vi "Init Phasor Explorer Settings.vi"(8 "error in (no error)":errorcluster) -> (0 "error out":errorcluster)   [LabVIEW 2019]
uses:
  Phasor Explorer Settings List.ctl
  Phasor Explorer Display Parameters.ctl
  Type of Series.ctl
  Phasor Explorer Phasor Parameters.ctl
  Phasor Calculation Type.ctl
  SEPL Type.ctl
  Phasor Explorer Decay Parameters.ctl
  IRF Model.ctl
  Phasor Explorer Gate Parameters.ctl
  Gate Type.ctl
  Type of User-defined Function.ctl
  Phasor Explorer Detector Parameters.ctl
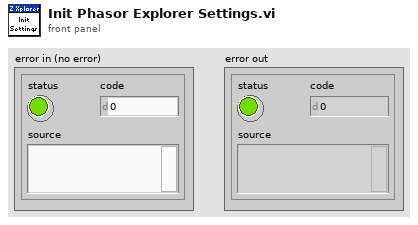
[diagram p1: front panel]
types:
  T1 = typedef "Phasor Explorer Settings List.ctl" = enum16{"Display Parameters", "Phasor Parameters", "Decay & IRF Parameters", "Gate Parameters", "Detector Parameters", "f*", "tau*"}
  T2 = typedef "Phasor Explorer Display Parameters.ctl" = cluster{"# Points":i32, "Ramp Type":enum16{"Linear", "Logarithmic"}, "Type of Series":T3, "Min tau":dbl[unit], "Max tau":dbl[unit], "Include 0":bool, "Include Infinity":bool}
  T3 = typedef "Type of Series.ctl" = enum16{"1-Exp Decays", "Linear Combination of 1-Exp"}
  T4 = typedef "Phasor Explorer Phasor Parameters.ctl" = cluster{"Harmonic Frequency":dbl[unit], "Use f* = 1/D Frequency":bool, "Calibrated Phasor":bool, "Calibration Lifetime":dbl[unit], "Phasor Calculation":T5, "SEPL Type":T6, "# Gates":dbl, "Square Gate Width":dbl[unit], "Show Ticks":bool}
  T5 = typedef "Phasor Calculation Type.ctl" = enum16{"Direct Sum", "Analytical Formula"}
  T6 = typedef "SEPL Type.ctl" = enum16{"UC", "L_N", "L_N[W]", "L_X"}
  T7 = typedef "Phasor Explorer Decay Parameters.ctl" = cluster{"Lifetime":dbl[unit], "IRF Offset":dbl[unit], "IRF Period":dbl[unit], "Normalized Decays":bool, "IRF Model":T8, "IRF Parameter 1":dbl[unit]}
  T8 = typedef "IRF Model.ctl" = enum16{"Dirac", "Exponential"}
  T9 = typedef "Phasor Explorer Gate Parameters.ctl" = cluster{"First Gate Start":dbl[unit], "Use Gate Center":bool, "Gate Width":dbl[unit], "Gate Step":dbl[unit], "# Gates":dbl, "Gate Type":T10, "Edge Width":dbl[unit], "Top Slope":dbl[unit], "Reversed Sawtooth?":bool, "Analytical Computation":bool, "Integration":enum32{"Item 0", "Item 1"}, "Tolerance":dbl, "# Steps":dbl, "Type of User-defined Function":T11, "Use Gate Step":bool}
  T10 = typedef "Gate Type.ctl" = enum16{"Square", "Finite Edge Square", "Finite Edge, Tilted Top Square", "Triangle", "Sawtooth", "User-defined"}
  T11 = typedef "Type of User-defined Function.ctl" = enum16{"Gate", "IRF"}
  T12 = typedef "Phasor Explorer Detector Parameters.ctl" = cluster{"Frames/Image":i32, "Gates/Frame":i32, "Bits/Frame":i32, "Multiplicity":i32, "Incident Signal":dbl, "Poisson Signal":bool}
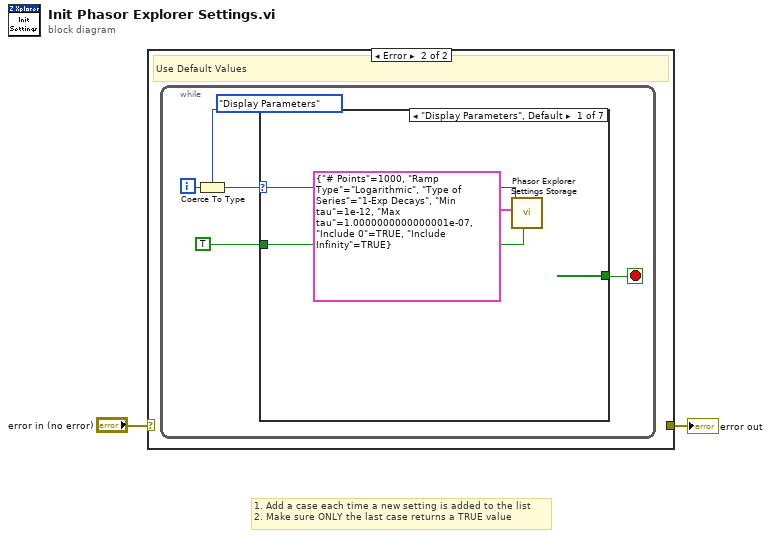
[diagram p0: block diagram]
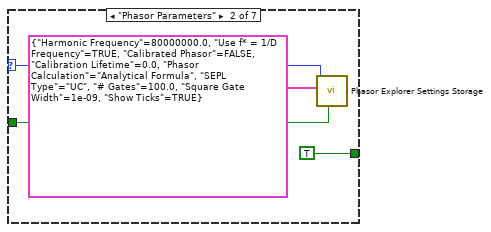
[diagram p3: hidden frame]
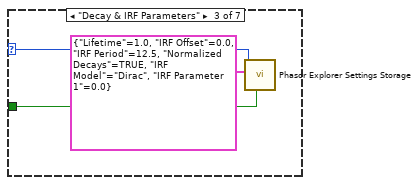
[diagram p4: hidden frame]
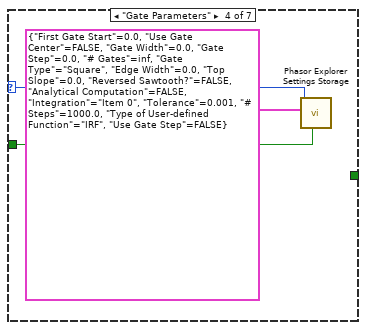
[diagram p5: hidden frame]
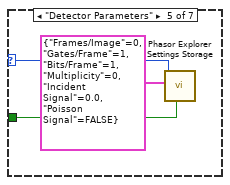
[diagram p6: hidden frame]
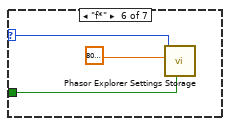
[diagram p7: hidden frame]
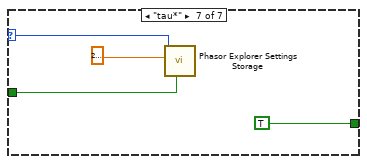
[diagram p8: hidden frame]
diagram:
  # "1. Add a case each time a new setting is added to the list\n2. Make sure ONLY the last case returns a TRUE value"
  n1 = case shown="Error" "error in (no error)" {
    selector: "error in (no error)" -> [w3 _]
    tunnel: [w3 _] -> w1
    frame No Error {
    }
    frame Error {
      # "Use Default Values"
      n2 = while {
        i -> [w8]
        stop <- w4 stop-if-true
        n3 = Coerce To Type(0:w8, 1:Phasor_Explorer_Settings_List."Display Parameters" ("PhXP Settings List")) -> (2:w6:T1)
        n4 = case shown="\"Display Parameters\", Default" w6 {
          selector: w6 -> [w11 w15 w18 w21 w24 w27 w31]
          tunnel: TRUE -> [w10 w13 w17 w20 w23 w26 w30]
          tunnel: [_ TRUE _ _ _ _ TRUE] -> w4
          frame "Display Parameters", Default {
            n5 = call "Phasor Explorer Settings Storage.vi"("Set/Get(F)"=w10, "Variant Data in"=T2 {"# Points"=1000, "Ramp Type"=enum."Logarithmic", "Type of Series"=enum."1-Exp Decays", "Min tau"=1e-12, "Max tau"=1.0000000000000001e-07, "Include 0"=TRUE, "Include Infinity"=TRUE} ("Phasor Explorer Display Parameters"), "Settings List"=w11) -> ()  [unwired: 7 in, 2 out]
          }
          frame "Phasor Parameters" {
            n6 = call "Phasor Explorer Settings Storage.vi"("Set/Get(F)"=w13, "Variant Data in"=T4 {"Harmonic Frequency"=80000000.0, "Use f* = 1/D Frequency"=TRUE, "Calibrated Phasor"=FALSE, "Calibration Lifetime"=0.0, "Phasor Calculation"=enum."Analytical Formula", "SEPL Type"=enum."UC", "# Gates"=100.0, "Square Gate Width"=1e-09, "Show Ticks"=TRUE} ("Phasor Explorer Phasor Parameters"), "Settings List"=w15) -> ()  [unwired: 7 in, 2 out]
          }
          frame "Decay & IRF Parameters" {
            n7 = call "Phasor Explorer Settings Storage.vi"("Set/Get(F)"=w17, "Variant Data in"=T7 {"Lifetime"=1.0, "IRF Offset"=0.0, "IRF Period"=12.5, "Normalized Decays"=TRUE, "IRF Model"=enum."Dirac", "IRF Parameter 1"=0.0} ("Phasor Explorer Decay Parameters"), "Settings List"=w18) -> ()  [unwired: 7 in, 2 out]
          }
          frame "Gate Parameters" {
            n8 = call "Phasor Explorer Settings Storage.vi"("Set/Get(F)"=w20, "Variant Data in"=T9 {"First Gate Start"=0.0, "Use Gate Center"=FALSE, "Gate Width"=0.0, "Gate Step"=0.0, "# Gates"=inf, "Gate Type"=enum."Square", "Edge Width"=0.0, "Top Slope"=0.0, "Reversed Sawtooth?"=FALSE, "Analytical Computation"=FALSE, "Integration"=enum."Item 0", "Tolerance"=0.001, "# Steps"=1000.0, "Type of User-defined Function"=enum."IRF", "Use Gate Step"=FALSE} ("Phasor Explorer Gate Parameters"), "Settings List"=w21) -> ()  [unwired: 7 in, 2 out]
          }
          frame "Detector Parameters" {
            n9 = call "Phasor Explorer Settings Storage.vi"("Set/Get(F)"=w23, "Variant Data in"=T12 {"Frames/Image"=0, "Gates/Frame"=1, "Bits/Frame"=1, "Multiplicity"=0, "Incident Signal"=0.0, "Poisson Signal"=FALSE} ("Phasor Explorer Detector Parameters"), "Settings List"=w24) -> ()  [unwired: 7 in, 2 out]
          }
          frame "f*" {
            n10 = call "Phasor Explorer Settings Storage.vi"("Set/Get(F)"=w26, "Variant Data in"=dbl[unit] 80000000.0 ("f0"), "Settings List"=w27) -> ()  [unwired: 7 in, 2 out]
          }
          frame "tau*" {
            n11 = call "Phasor Explorer Settings Storage.vi"("Set/Get(F)"=w30, "Variant Data in"=dbl[unit] 2e-09 ("f0"), "Settings List"=w31) -> ()  [unwired: 7 in, 2 out]
          }
        }
      }
    }
  }
  "error out" <- w1
